vi "matchingLocales.vi"(6 "country (AnyCountry)":T1 items=["AnyCountry", "Afghanistan", "Albania", "Algeria", "AmericanSamoa", "Andorra", "Angola", "Anguilla", "Antarctica", "AntiguaAndBarbuda", "Argentina", "Armenia", "Aruba", "Australia", "Austria", "Azerbaijan", "Bahamas", "Bahrain", "Bangladesh", "Barbados", "Belarus", "Belgium", "Belize", "Benin", "Bermuda", "Bhutan", "Bolivia", "BosniaAndHerzegowina", "Botswana", "BouvetIsland", "Brazil", "BritishIndianOceanTerritory", "Brunei", "Bulgaria", "BurkinaFaso", "Burundi", "Cambodia", "Cameroon", "Canada", "CapeVerde", "CaymanIslands", "CentralAfricanRepublic", "Chad", "Chile", "China", "ChristmasIsland", "CocosIslands", "Colombia", "Comoros", "CongoKinshasa", "CongoBrazzaville", "CookIslands", "CostaRica", "IvoryCoast", "Croatia", "Cuba", "Cyprus", "CzechRepublic", "Denmark", "Djibouti", "Dominica", "DominicanRepublic", "EastTimor", "Ecuador", "Egypt", "ElSalvador", "EquatorialGuinea", "Eritrea", "Estonia", "Ethiopia", "FalklandIslands", "FaroeIslands", "Fiji", "Finland", "France", "Guernsey", "FrenchGuiana", "FrenchPolynesia", "FrenchSouthernTerritories", "Gabon", "Gambia", "Georgia", "Germany", "Ghana", "Gibraltar", "Greece", "Greenland", "Grenada", "Guadeloupe", "Guam", "Guatemala", "Guinea", "GuineaBissau", "Guyana", "Haiti", "HeardAndMcDonaldIslands", "Honduras", "HongKong", "Hungary", "Iceland", "India", "Indonesia", "Iran", "Iraq", "Ireland", "Israel", "Italy", "Jamaica", "Japan", "Jordan", "Kazakhstan", "Kenya", "Kiribati", "NorthKorea", "SouthKorea", "Kuwait", "Kyrgyzstan", "Laos", "Latvia", "Lebanon", "Lesotho", "Liberia", "Libya", "Liechtenstein", "Lithuania", "Luxembourg", "Macau", "Macedonia", "Madagascar", "Malawi", "Malaysia", "Maldives", "Mali", "Malta", "MarshallIslands", "Martinique", "Mauritania", "Mauritius", "Mayotte", "Mexico", "Micronesia", "Moldova", "Monaco", "Mongolia", "Montserrat", "Morocco", "Mozambique", "Myanmar", "Namibia", "NauruCountry", "Nepal", "Netherlands", "CuraSao", "NewCaledonia", "NewZealand", "Nicaragua", "Niger", "Nigeria", "Niue", "NorfolkIsland", "NorthernMarianaIslands", "Norway", "Oman", "Pakistan", "Palau", "PalestinianTerritories", "Panama", "PapuaNewGuinea", "Paraguay", "Peru", "Philippines", "Pitcairn", "Poland", "Portugal", "PuertoRico", "Qatar", "Reunion", "Romania", "Russia", "Rwanda", "SaintKittsAndNevis", "SaintLucia", "SaintVincentAndTheGrenadines", "Samoa", "SanMarino", "SaoTomeAndPrincipe", "SaudiArabia", "Senegal", "Seychelles", "SierraLeone", "Singapore", "Slovakia", "Slovenia", "SolomonIslands", "Somalia", "SouthAfrica", "SouthGeorgiaAndTheSouthSandwichIslands", "Spain", "SriLanka", "SaintHelena", "SaintPierreAndMiquelon", "Sudan", "Suriname", "SvalbardAndJanMayenIslands", "Swaziland", "Sweden", "Switzerland", "Syria", "Taiwan", "Tajikistan", "Tanzania", "Thailand", "Togo", "TokelauCountry", "Tonga", "TrinidadAndTobago", "Tunisia", "Turkey", "Turkmenistan", "TurksAndCaicosIslands", "TuvaluCountry", "Uganda", "Ukraine", "UnitedArabEmirates", "UnitedKingdom", "UnitedStates", "UnitedStatesMinorOutlyingIslands", "Uruguay", "Uzbekistan", "Vanuatu", "VaticanCityState", "Venezuela", "Vietnam", "BritishVirginIslands", "UnitedStatesVirginIslands", "WallisAndFutunaIslands", "WesternSahara", "Yemen", "CanaryIslands", "Zambia", "Zimbabwe", "ClippertonIsland", "Montenegro", "Serbia", "SaintBarthelemy", "SaintMartin", "LatinAmerica", "AscensionIsland", "AlandIslands", "DiegoGarcia", "CeutaAndMelilla", "IsleOfMan", "Jersey", "TristanDaCunha", "SouthSudan", "Bonaire", "SintMaarten", "Kosovo", "EuropeanUnion", "OutlyingOceania", "World", "Europe"], 8 "Error In":errorcluster, 9 "script (AnyScript)":T2 items=["AnyScript", "ArabicScript", "CyrillicScript", "DeseretScript", "GurmukhiScript", "SimplifiedHanScript", "TraditionalHanScript", "LatinScript", "MongolianScript", "TifinaghScript", "ArmenianScript", "BengaliScript", "CherokeeScript", "DevanagariScript", "EthiopicScript", "GeorgianScript", "GreekScript", "GujaratiScript", "HebrewScript", "JapaneseScript", "KhmerScript", "KannadaScript", "KoreanScript", "LaoScript", "MalayalamScript", "MyanmarScript", "OriyaScript", "TamilScript", "TeluguScript", "ThaanaScript", "ThaiScript", "TibetanScript", "SinhalaScript", "SyriacScript", "YiScript", "VaiScript", "AvestanScript", "BalineseScript", "BamumScript", "BatakScript", "BopomofoScript", "BrahmiScript", "BugineseScript", "BuhidScript", "CanadianAboriginalScript", "CarianScript", "ChakmaScript", "ChamScript", "CopticScript", "CypriotScript", "EgyptianHieroglyphsScript", "FraserScript", "GlagoliticScript", "GothicScript", "HanScript", "HangulScript", "HanunooScript", "ImperialAramaicScript", "InscriptionalPahlaviScript", "InscriptionalParthianScript", "JavaneseScript", "KaithiScript", "KatakanaScript", "KayahLiScript", "KharoshthiScript", "LannaScript", "LepchaScript", "LimbuScript", "LinearBScript", "LycianScript", "LydianScript", "MandaeanScript", "MeiteiMayekScript", "MeroiticScript", "MeroiticCursiveScript", "NkoScript", "NewTaiLueScript", "OghamScript", "OlChikiScript", "OldItalicScript", "OldPersianScript", "OldSouthArabianScript", "OrkhonScript", "OsmanyaScript", "PhagsPaScript", "PhoenicianScript", "PollardPhoneticScript", "RejangScript", "RunicScript", "SamaritanScript", "SaurashtraScript", "SharadaScript", "ShavianScript", "SoraSompengScript", "CuneiformScript", "SundaneseScript", "SylotiNagriScript", "TagalogScript", "TagbanwaScript", "TaiLeScript", "TaiVietScript", "TakriScript", "UgariticScript", "BrailleScript", "HiraganaScript", "CaucasianAlbanianScript", "BassaVahScript", "DuployanScript", "ElbasanScript", "GranthaScript", "PahawhHmongScript", "KhojkiScript", "LinearAScript", "MahajaniScript", "ManichaeanScript", "MendeKikakuiScript", "ModiScript", "MroScript", "OldNorthArabianScript", "NabataeanScript", "PalmyreneScript", "PauCinHauScript", "OldPermicScript", "PsalterPahlaviScript", "SiddhamScript", "KhudawadiScript", "TirhutaScript", "VarangKshitiScript", "AhomScript", "AnatolianHieroglyphsScript", "HatranScript", "MultaniScript", "OldHungarianScript", "SignWritingScript", "AdlamScript", "BhaiksukiScript", "MarchenScript", "NewaScript", "OsageScript", "TangutScript", "HanWithBopomofoScript", "JamoScript"], 10 "language (AnyLanguage)":T3 items=["AnyLanguage", "C", "Abkhazian", "Oromo", "Afar", "Afrikaans", "Albanian", "Amharic", "Arabic", "Armenian", "Assamese", "Aymara", "Azerbaijani", "Bashkir", "Basque", "Bengali", "Dzongkha", "Bihari", "Bislama", "Breton", "Bulgarian", "Burmese", "Belarusian", "Khmer", "Catalan", "Chinese", "Corsican", "Croatian", "Czech", "Danish", "Dutch", "English", "Esperanto", "Estonian", "Faroese", "Fijian", "Finnish", "French", "WesternFrisian", "Gaelic", "Galician", "Georgian", "German", "Greek", "Greenlandic", "Guarani", "Gujarati", "Hausa", "Hebrew", "Hindi", "Hungarian", "Icelandic", "Indonesian", "Interlingua", "Interlingue", "Inuktitut", "Inupiak", "Irish", "Italian", "Japanese", "Javanese", "Kannada", "Kashmiri", "Kazakh", "Kinyarwanda", "Kirghiz", "Korean", "Kurdish", "Rundi", "Lao", "Latin", "Latvian", "Lingala", "Lithuanian", "Macedonian", "Malagasy", "Malay", "Malayalam", "Maltese", "Maori", "Marathi", "Marshallese", "Mongolian", "NauruLanguage", "Nepali", "NorwegianBokmal", "Occitan", "Oriya", "Pashto", "Persian", "Polish", "Portuguese", "Punjabi", "Quechua", "Romansh", "Romanian", "Russian", "Samoan", "Sango", "Sanskrit", "Serbian", "Ossetic", "SouthernSotho", "Tswana", "Shona", "Sindhi", "Sinhala", "Swati", "Slovak", "Slovenian", "Somali", "Spanish", "Sundanese", "Swahili", "Swedish", "Sardinian", "Tajik", "Tamil", "Tatar", "Telugu", "Thai", "Tibetan", "Tigrinya", "Tongan", "Tsonga", "Turkish", "Turkmen", "Tahitian", "Uighur", "Ukrainian", "Urdu", "Uzbek", "Vietnamese", "Volapuk", "Welsh", "Wolof", "Xhosa", "Yiddish", "Yoruba", "Zhuang", "Zulu", "NorwegianNynorsk", "Bosnian", "Divehi", "Manx", "Cornish", "Akan", "Konkani", "Ga", "Igbo", "Kamba", "Syriac", "Blin", "Geez", "Koro", "Sidamo", "Atsam", "Tigre", "Jju", "Friulian", "Venda", "Ewe", "Walamo", "Hawaiian", "Tyap", "Nyanja", "Filipino", "SwissGerman", "SichuanYi", "Kpelle", "LowGerman", "SouthNdebele", "NorthernSotho", "NorthernSami", "Taroko", "Gusii", "Taita", "Fulah", "Kikuyu", "Samburu", "Sena", "NorthNdebele", "Rombo", "Tachelhit", "Kabyle", "Nyankole", "Bena", "Vunjo", "Bambara", "Embu", "Cherokee", "Morisyen", "Makonde", "Langi", "Ganda", "Bemba", "Kabuverdianu", "Meru", "Kalenjin", "Nama", "Machame", "Colognian", "Masai", "Soga", "Luyia", "Asu", "Teso", "Saho", "KoyraChiini", "Rwa", "Luo", "Chiga", "CentralMoroccoTamazight", "KoyraboroSenni", "Shambala", "Bodo", "Avaric", "Chamorro", "Chechen", "Church", "Chuvash", "Cree", "Haitian", "Herero", "HiriMotu", "Kanuri", "Komi", "Kongo", "Kwanyama", "Limburgish", "LubaKatanga", "Luxembourgish", "Navaho", "Ndonga", "Ojibwa", "Pali", "Walloon", "Aghem", "Basaa", "Zarma", "Duala", "JolaFonyi", "Ewondo", "Bafia", "MakhuwaMeetto", "Mundang", "Kwasio", "Nuer", "Sakha", "Sangu", "CongoSwahili", "Tasawaq", "Vai", "Walser", "Yangben", "Avestan", "Asturian", "Ngomba", "Kako", "Meta", "Ngiemboon", "Aragonese", "Akkadian", "AncientEgyptian", "AncientGreek", "Aramaic", "Balinese", "Bamun", "BatakToba", "Buginese", "Buhid", "Carian", "Chakma", "ClassicalMandaic", "Coptic", "Dogri", "EasternCham", "EasternKayah", "Etruscan", "Gothic", "Hanunoo", "Ingush", "LargeFloweryMiao", "Lepcha", "Limbu", "Lisu", "Lu", "Lycian", "Lydian", "Mandingo", "Manipuri", "Meroitic", "NorthernThai", "OldIrish", "OldNorse", "OldPersian", "OldTurkish", "Pahlavi", "Parthian", "Phoenician", "PrakritLanguage", "Rejang", "Sabaean", "Samaritan", "Santali", "Saurashtra", "Sora", "Sylheti", "Tagbanwa", "TaiDam", "TaiNua", "Ugaritic", "Akoose", "Lakota", "StandardMoroccanTamazight", "Mapuche", "CentralKurdish", "LowerSorbian", "UpperSorbian", "Kenyang", "Mohawk", "Nko", "Prussian", "Kiche", "SouthernSami", "LuleSami", "InariSami", "SkoltSami", "Warlpiri", "ManichaeanMiddlePersian", "Mende", "AncientNorthArabian", "LinearA", "HmongNjua", "Ho", "Lezghian", "Bassa", "Mono", "TedimChin", "Maithili", "Ahom", "AmericanSignLanguage", "ArdhamagadhiPrakrit", "Bhojpuri", "HieroglyphicLuwian", "LiteraryChinese", "Mazanderani", "Mru", "Newari", "NorthernLuri", "Palauan", "Papiamento", "Saraiki", "TokelauLanguage", "TokPisin", "TuvaluLanguage", "UncodedLanguages", "Cantonese", "Osage", "Tangut"]) -> (0 "Error Out":errorcluster, 2 "Value":refnum<class "QLocale.lvclass">[](array[class]))   [LabVIEW 2014, in "QLocale.lvclass"]
doc: "LabVIEW-specific documentation is not yet available. See <b>https://doc.qt.io/qt-5/qlocale.html#matchingLocales</b>"
uses:
  QLocale.lvclass
  Language.ctl
  Script.ctl
  Country.ctl
  LQSerialData/LQSerialData.lvclass/LQSerialData.ctl
  LQ Core.lvlib
  LQSerialData/LQSerialData.lvclass
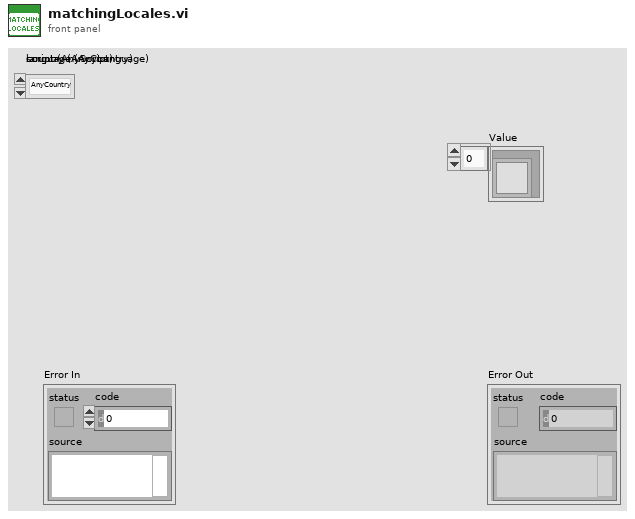
[diagram p1: front panel]
types:
  T1 = typedef "QLocale.lvclass/Country.ctl" = i32
  T2 = typedef "QLocale.lvclass/Script.ctl" = i32
  T3 = typedef "QLocale.lvclass/Language.ctl" = i32
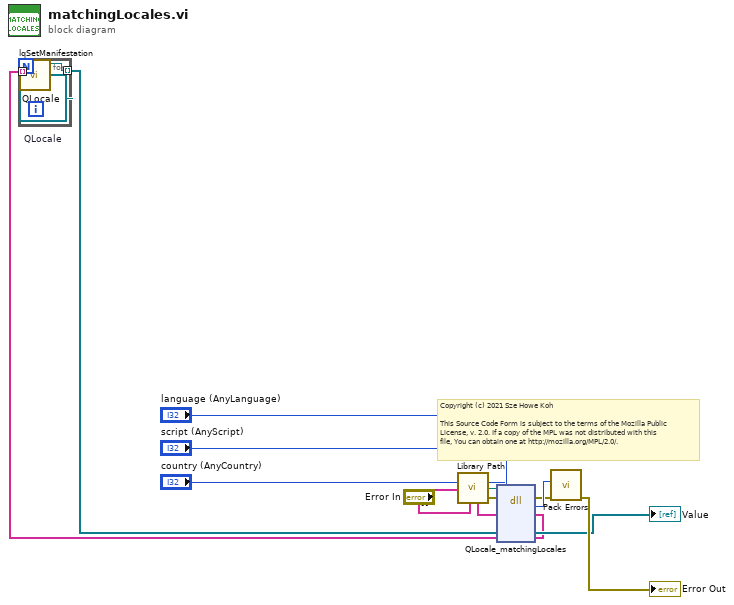
[diagram p0: block diagram]
diagram:
  # "Copyright (c) 2021 Sze Howe Koh\n\nThis Source Code Form is subject to the terms of the Mozilla Public\nLicense, v. 2.0. If a copy of the MPL was not distributed with this\nfile, You can obtain one at http://mozilla.org/MPL/2.0/."
  n1 = call "Library Path.vi"() -> ("Library Path"=w9:path)
  n2 = dll-call lib="?" fn="QLocale_matchingLocales"(path in=w9, error in="Error In", "_retVal"=string[] [] ("retVal"), "language"="language (AnyLanguage)", "script"="script (AnyScript)", "country"="country (AnyCountry)") -> (error out=w7:errorcluster, w8:i32, "_retVal"=w4:string[])  [unwired: 4 in, 1 out]
  n3 = for {
    tunnel: [w14] -> w5 mode=indexing
    tunnel: w4 -> [w12] mode=indexing
    w13 = refnum<class "QLocale.lvclass"> refnum  # QLocale
    n4 = call "lqSetManifestation.vi"("Manifestation"=w12, "LQSerialData in"=w13) -> ("LQSerialData out"=w14:refnum<class "QLocale.lvclass">)  [unwired: 8 in, 1 out]
  }
  "Value" <- w5
  n5 = call "Pack Errors.vi"("Error In"=w7, "Error Code"=w8) -> ("Error Out"=→"Error Out":errorcluster)  [unwired: 9 in]
